vi "ECG_final.vi"() -> ()   [LabVIEW 2021]
panel:
  out "Heart Failure":bool
  in  "SAVE":bool
  out "BPMs":dbl
  out "Propanolol":bool
  out "Atropina":bool
  out "R Wave Detected":bool
  out "Pacemaker":bool
  in  "Sampling Rate (S/s)":u16(ring) items=["25", "50", "100", "200"]
  in  "Upper Limit":dbl
  in  "Lower Limit":dbl
  out "String":string
  in  "Começar":bool
  out "Waveform Chart":u8(graph)
  out "error out":errorcluster
  in  "stop":bool
  in  "Clear":bool
  out "Comunication":string
  in  "error in (no error)":errorcluster
  in  "VISA resource name":refnum<visa-resource-name>="COM4"
  # "Data aquisition setup"
  # "Patient Information"
  # "TERMS AND CONDITIONS OF USE"
  # "Montanex warrants to Buyer that Products manufactured by Montanex that are sold to Buyer will be possibly free from defects in material and workmanship under normal use for the following warranty periods: (i) 6 months following shipment from Montanex in the case of consumables;  \n\nAll Montanex Buyers and Users agree to the following:\nMontanex cannot be held responsible for any bodily harm that may come to Montanex Buyers and Users while operating or being subjected to any tests by any Montanex devices;\n\nBy agreeing to operate or be subjected to any tests by this or any Montanex device you are agreeing to rate it a 20 out of 20 in any evaluations this or any Montanex device may be subjected to; \n\nFailure to comply with the agreed terms and conditions will be met with legal action."
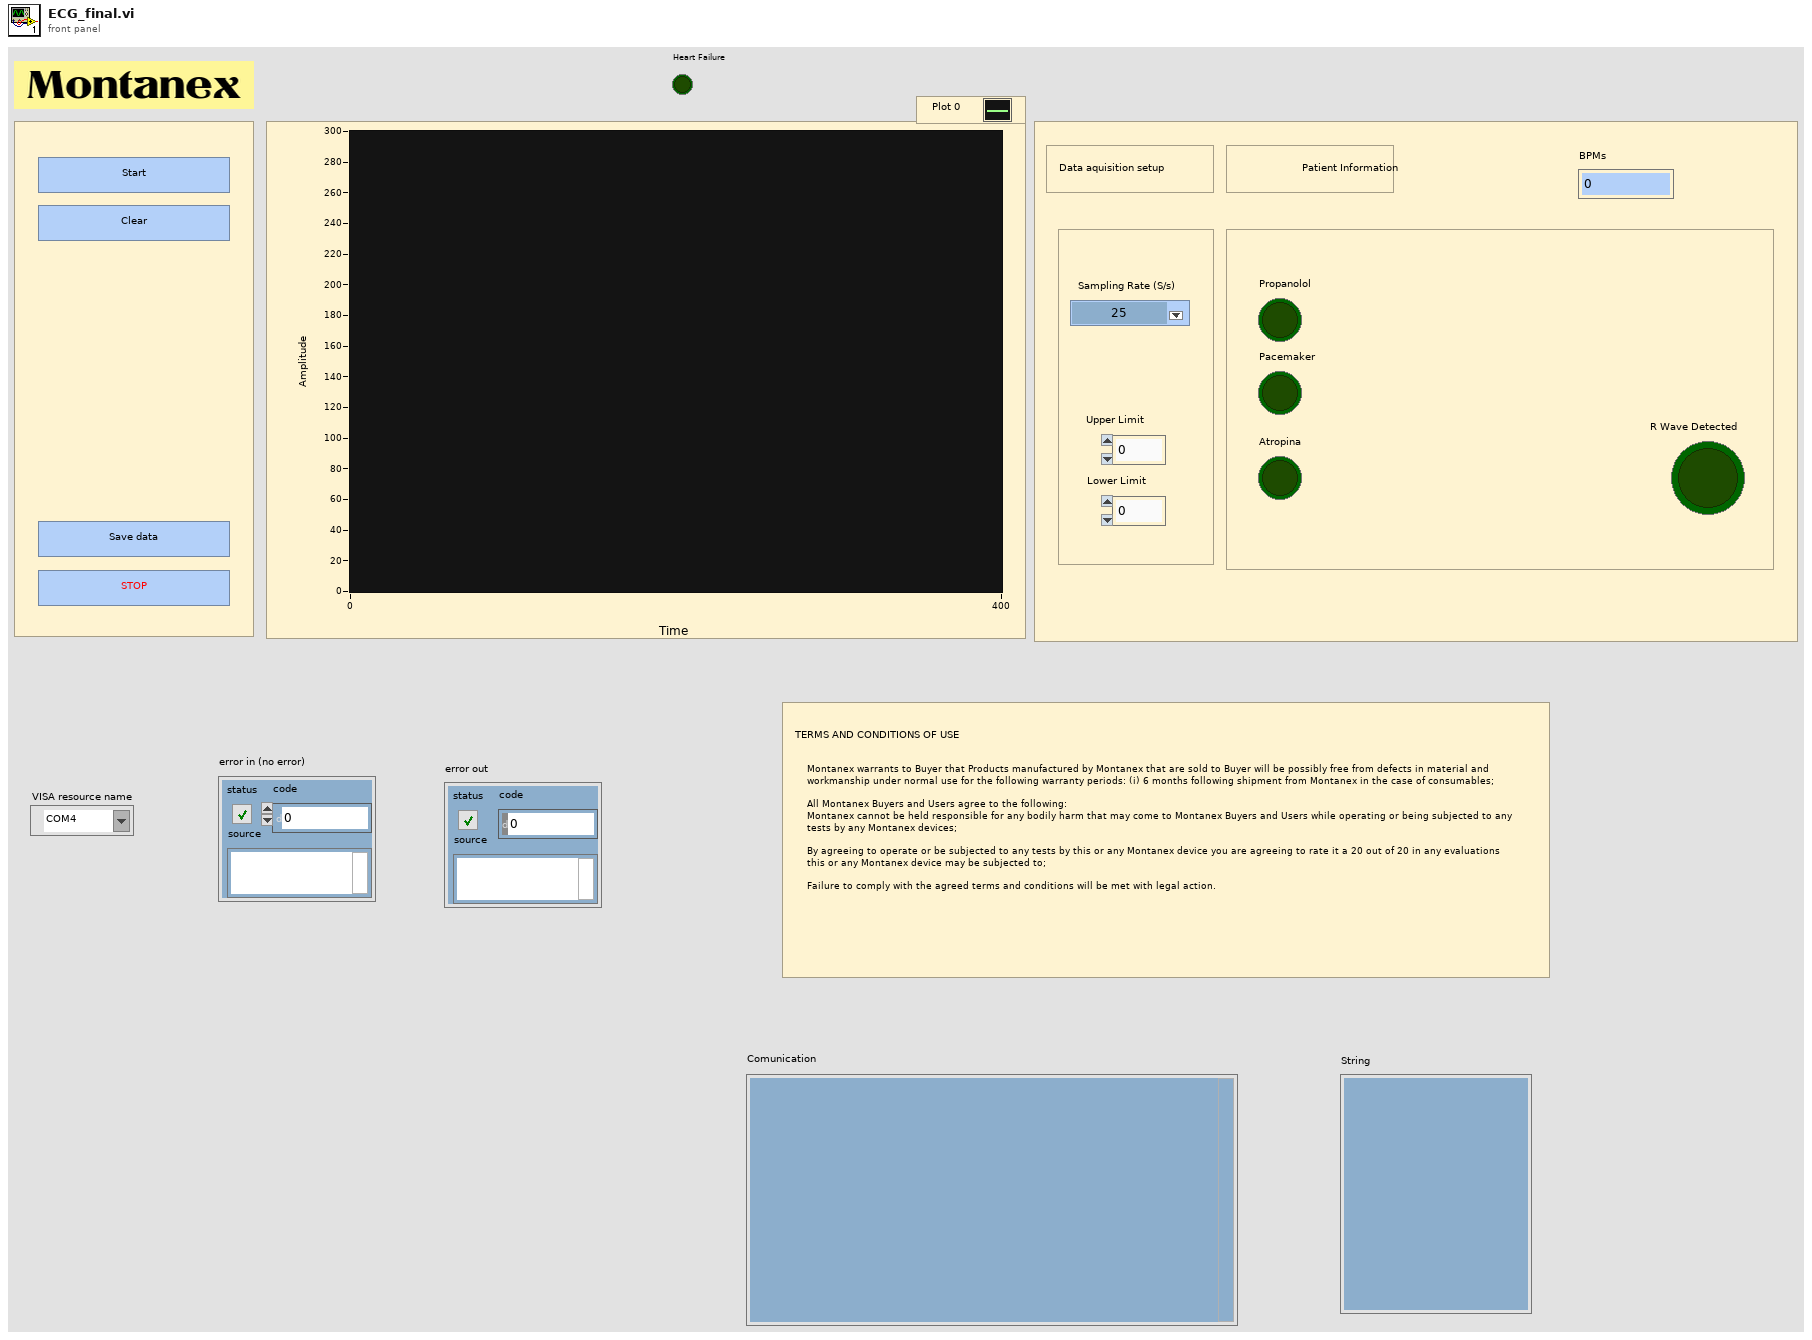
[diagram p1: front panel]
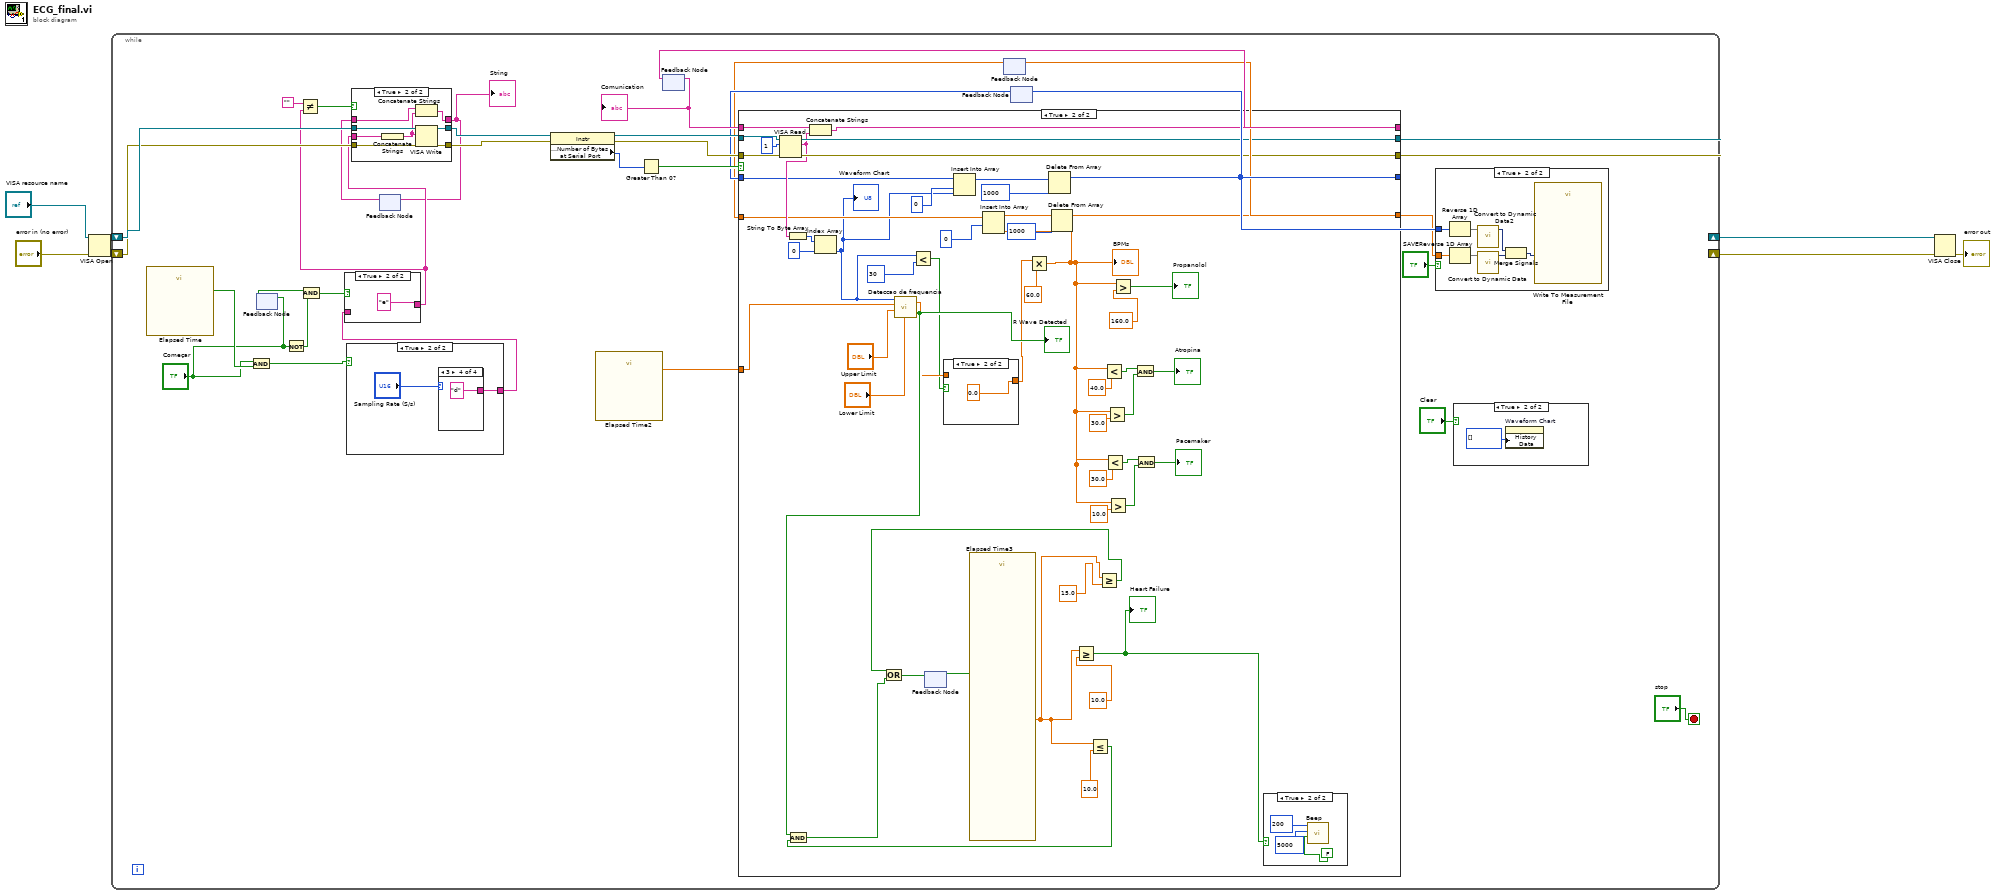
[diagram p0: block diagram]
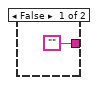
[diagram p5: hidden frame]
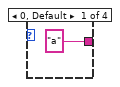
[diagram p6: hidden frame]
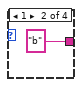
[diagram p7: hidden frame]
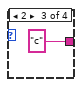
[diagram p8: hidden frame]
diagram:
  n1 = VISA Open(error in (no error)="error in (no error)", VISA resource name="VISA resource name") -> (VISA resource name=w5:refnum<visa-resource-name>, error out=w4:errorcluster)  [unwired: 3 in]
  n2 = while {
    shift-right: [w33] -> w3
    shift-left: w5 -> [w31]
    shift-right: [w32] -> w2
    shift-left: w4 -> [w29]
    stop <- "stop" stop-if-true
    n3 = call "Elapsed Time"() -> ("Time has Elapsed"=w24:bool)  [unwired: 12 in, 7 out]
    n4 = And(x="Começar", y=w24) -> (x .and. y?=w23:bool)
    n5 = feedback-in #1("Começar") -> ()
    n6 = feedback #1() -> (w20:bool)  [unwired: 1 in]
    n7 = Not(x="Começar") -> (.not. x?=w19:bool)
    n8 = And(x=w20, y=w19) -> (x .and. y?=w17:bool)
    n9 = case shown="True" w23 {
      tunnel: ["" w51] -> w22
      frame False {
      }
      frame True {
        n10 = case shown="3" "Sampling Rate (S/s)" {
          tunnel: ["a" "b" "c" "d"] -> w51
          frame 0, Default {
          }
          frame 1 {
          }
          frame 2 {
          }
          frame 3 {
          }
        }
      }
    }
    n11 = case shown="True" w17 {
      tunnel: w22 -> [w48 _]
      tunnel: [w48 "e"] -> w21
      frame False {
      }
      frame True {
      }
    }
    n12 = Not Equal?(x="", y=w21) -> (x != y?=w26:bool)
    n13 = feedback #2() -> (w15:string)  [unwired: 1 in]
    n14 = case shown="True" w26 {
      tunnel: w31 -> [w59 w67]
      tunnel: [w59 w66] -> w30
      tunnel: w29 -> [w58 w65]
      tunnel: [w58 w64] -> w28
      tunnel: w21 -> [_ w63]
      tunnel: [w57 w61] -> w16
      tunnel: w15 -> [w57 w60]
      frame False {
      }
      frame True {
        n15 = Concatenate Strings(w63) -> (w62:string)
        n16 = Concatenate Strings(w60, w62) -> (w61:string)
        n17 = VISA Write(VISA resource name=w67, write buffer=w62, error in (no error)=w65) -> (VISA resource name out=w66:refnum<visa-resource-name>, error out=w64:errorcluster)  [unwired: 1 out]
      }
    }
    "String" <- w16
    n18 = feedback-in #2(w16) -> ()
    n19 = property class="Instr"(reference=w30, error in=w28) -> (reference out=w36:refnum<visa-resource-name>, error out=w35:errorcluster, "Serial Settings:Number of Bytes at Serial Port"=w38:u32)
    n20 = call "Elapsed Time2"() -> ("Elapsed Time (s)"=w25:dbl)  [unwired: 12 in, 7 out]
    n21 = Greater Than 0?(x=w38) -> (x > 0?=w37:bool)
    n22 = feedback #3() -> (w34:string)  [unwired: 1 in]
    "Comunication" <- w34
    n23 = feedback #4() -> (w10:dbl[])  [unwired: 1 in]
    n24 = feedback #5() -> (w14:u8[])  [unwired: 1 in]
    n25 = case shown="True" w37 {
      tunnel: w36 -> [w72 w124]
      tunnel: w35 -> [w71 w125]
      tunnel: [w72 w122] -> w33
      tunnel: [w71 w121] -> w32
      tunnel: [w70 w119] -> w11
      tunnel: w34 -> [w70 w120]
      tunnel: w25 -> [_ w118]
      tunnel: [w69 w99] -> w9
      tunnel: w14 -> [w69 w98]
      tunnel: w10 -> [w68 w93]
      tunnel: [w68 w91] -> w8
      frame False {
      }
      frame True {
        n26 = VISA Read(VISA resource name=w124, byte count=u32 1, error in (no error)=w125) -> (VISA resource name out=w122:refnum<visa-resource-name>, read buffer=w103:string, error out=w121:errorcluster)  [unwired: 1 out]
        n27 = String To Byte Array(string=w103) -> (unsigned byte array=w101:u8[])
        n28 = Concatenate Strings(w120, w103) -> (w119:string)
        n29 = Index Array(array=w101, index=0) -> (element=w75:u8)
        "Waveform Chart" <- w75
        n30 = call "Deteccao de frequencia.vi"("Limiar inferior de deteccao"="Lower Limit", "Limiar superior de deteccao"="Upper Limit", "Tempo (s)"=w118, "Medida do sinal"=w75) -> ("Deteccao de limiar"=w80:bool, "Frequencia (Hz)"=w78:dbl)
        "R Wave Detected" <- w80
        n31 = Less?(x=w75, y=u8 30) -> (x < y?=w73:bool)
        n32 = feedback #6() -> (w82:bool)  [unwired: 1 in]
        n33 = case shown="True" w73 {
          tunnel: w78 -> [w126 _]
          tunnel: [w126 0.0] -> w77
          frame False {
          }
          frame True {
          }
        }
        n34 = Insert Into Array(array=w98, index=0, new element=w75) -> (w100:u8[])
        n35 = call "Elapsed Time3"("Reset"=w82) -> ("Elapsed Time (s)"=w87:dbl)  [unwired: 11 in, 7 out]
        n36 = Multiply(x=w77, y=60.0) -> (x*y=w90:dbl)
        "BPMs" <- w90
        n37 = Insert Into Array(array=w93, index=0, new element=w90) -> (w92:dbl[])
        n38 = Delete From Array(array=w100, index=1000) -> (array with subset deleted=w99:u8[])  [unwired: 1 in, 1 out]
        n39 = Delete From Array(array=w92, index=1000) -> (array with subset deleted=w91:dbl[])  [unwired: 1 in, 1 out]
        n40 = Greater Or Equal?(x=w87, y=10.0) -> (x >= y?=w79:bool)
        "Heart Failure" <- w79
        n41 = Less Or Equal?(x=w87, y=10.0) -> (x <= y?=w85:bool)
        n42 = And(x=w80, y=w85) -> (x .and. y?=w84:bool)
        n43 = Greater Or Equal?(x=w87, y=15.0) -> (x >= y?=w81:bool)
        n44 = Or(x=w81, y=w84) -> (x .or. y?=w83:bool)
        n45 = feedback-in #6(w83) -> ()
        n46 = Less?(x=w90, y=40.0) -> (x < y?=w111:bool)
        n47 = Less?(x=w90, y=30.0) -> (x < y?=w106:bool)
        n48 = Greater?(x=w90, y=30.0) -> (0:w110:bool)
        n49 = Greater?(x=w90, y=10.0) -> (0:w105:bool)
        n50 = Greater?(x=w90, y=160.0) -> (0:→"Propanolol":bool)
        n51 = And(x=w111, y=w110) -> (x .and. y?=→"Atropina":bool)
        n52 = And(x=w106, y=w105) -> (x .and. y?=→"Pacemaker":bool)
        n53 = case shown="True" w79 {
          frame False {
          }
          frame True {
            n54 = call <vilib>:"Beep.vi"("use system alert? (T)"=FALSE, "duration (msec)"=5000, "frequency (Hz)"=200) -> ()  [unwired: 9 in]
          }
        }
      }
    }
    n55 = feedback-in #3(w11) -> ()
    n56 = feedback-in #4(w8) -> ()
    n57 = feedback-in #5(w9) -> ()
    n58 = case shown="True" "SAVE" {
      tunnel: w9 -> [_ w47]
      tunnel: w8 -> [_ w46]
      frame False {
      }
      frame True {
        n59 = Reverse 1D Array(array=w47) -> (reversed array=w43:u8[])
        n60 = Reverse 1D Array(array=w46) -> (reversed array=w45:dbl[])
        n61 = call "Convert to Dynamic Data2"("Array"=w43) -> ("Dynamic Data Type"=w42:dynamicdata)  [unwired: 3 in]
        n62 = call "Convert to Dynamic Data"("Array"=w45) -> ("Dynamic Data Type"=w44:dynamicdata)  [unwired: 3 in]
        n63 = Merge Signals(w42, w44) -> (w41:dynamicdata)
        n64 = call "Write To Measurement File"("Signals"=w41) -> ()  [unwired: 16 in, 3 out]
      }
    }
    n65 = case shown="True" "Clear" {
      frame False {
      }
      frame True {
        n66 = property on="Waveform Chart" class="WFChart (strict)"("History Data"=u8[] []) -> ()  [unwired: 2 in, 2 out]
      }
    }
  }
  n67 = VISA Close(VISA resource name=w3, error in (no error)=w2) -> (error out=→"error out":errorcluster)
